vi "Append text file.vi"(8 "error in":errorcluster, 10 "text to write":string, 11 "file path (use dialog)":path) -> (0 "error out":errorcluster)   [LabVIEW 2013]
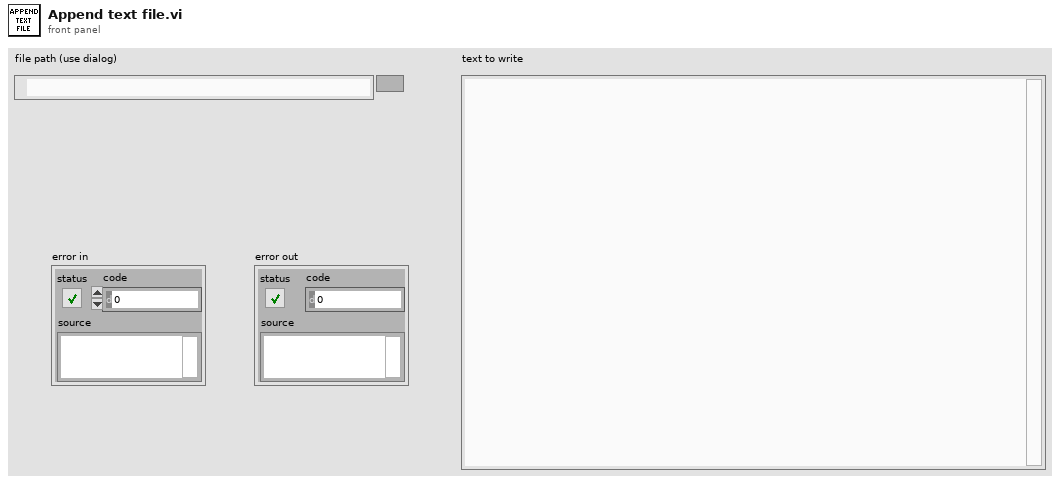
[diagram p1: front panel]
types:
  T1 = enum16{"open", "replace", "create", "open or create", "replace or create", "replace or create with confirmation"}
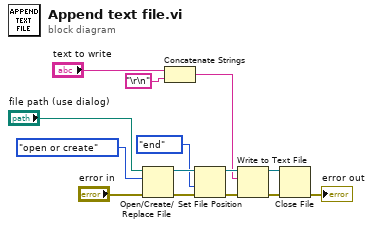
[diagram p0: block diagram]
diagram:
  n1 = Open/Create/Replace File(file path (use dialog)="file path (use dialog)", error in="error in", operation (0:open)=T1."open or create") -> (refnum out=w11:refnum<file>, error out=w9:errorcluster)  [unwired: 3 in, 1 out]
  n2 = Concatenate Strings("text to write", "\r\n") -> (w1:string)
  n3 = Set File Position(refnum=w11, from (0:start)=enum16{"start", "end", "current"}."end", error in=w9) -> (refnum out=w7:refnum<file>, error out=w8:errorcluster)  [unwired: 1 in]
  n4 = Write to Text File(file (use dialog)=w7, text=w1, error in=w8) -> (refnum out=w6:refnum<file>, error out=w5:errorcluster)  [unwired: 1 in, 1 out]
  n5 = Close File(refnum=w6, error in=w5) -> (error out=→"error out":errorcluster)  [unwired: 1 out]
